vi "Configure Offset and Limits (Reflection Measurement).vi"(0 "VISA resource name":refnum<visa-resource-name>, 1 "Limit Line Value (0 dBm)":dbl, 5 "Line Number (1: Line 1)":i32(ring)=1 items=["Line 1"=1, "Line 2"=2], 9 "Limit Type (0: Upper Line)":i32(ring) items=["Upper Line", "Lower Line"], 11 "error in (no error)":errorcluster) -> (4 "VISA resource name out":refnum<visa-resource-name>, 15 "error out":errorcluster)   [LabVIEW 2022 SP3, in "Agilent N934X Series.lvlib"]
doc: "Configures the general setting for offset and limits of reflection Measurement Option.\n\nNote:\nThis VI is only applicable for N9321C, N9322C, N9323C, N9324C models."
uses:
  <instrlib>/Agilent N934X Series/Agilent N934X Series.lvlib
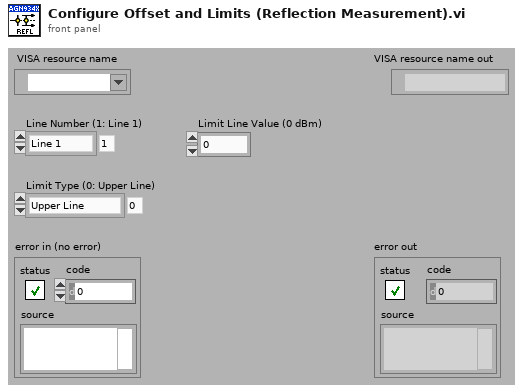
[diagram p1: front panel]
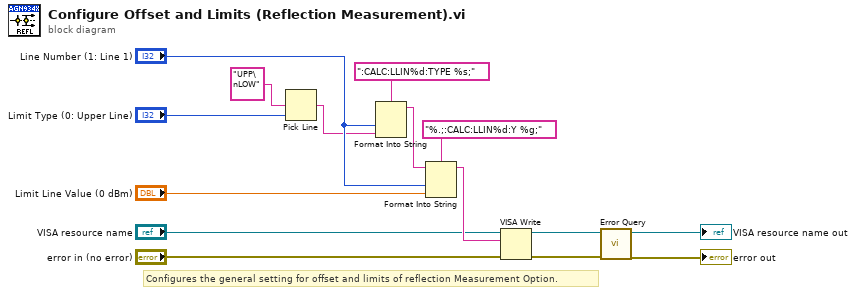
[diagram p0: block diagram]
diagram:
  # "Configures the general setting for offset and limits of reflection Measurement Option."
  n1 = Pick Line(multi-line string="UPP\nLOW", line index="Limit Type (0: Upper Line)") -> (output string=w11:string)  [unwired: 1 in]
  n2 = Format Into String(format string=":CALC:LLIN%d:TYPE %s;", "Line Number (1: Line 1)", w11) -> (resulting string=w10:string)  [unwired: 2 in, 1 out]
  n3 = Format Into String(format string="%.;:CALC:LLIN%d:Y %g;", initial string=w10, "Line Number (1: Line 1)", "Limit Line Value (0 dBm)") -> (resulting string=w7:string)  [unwired: 1 in, 1 out]
  n4 = VISA Write(VISA resource name="VISA resource name", write buffer=w7, error in (no error)="error in (no error)") -> (VISA resource name out=w4:refnum<visa-resource-name>, error out=w3:errorcluster)  [unwired: 1 out]
  n5 = call <instrlib>:"Error Query.vi"("error in (no error)"=w3, "VISA resource name"=w4) -> ("error out"=→"error out":errorcluster, "VISA resource name out"=→"VISA resource name out":refnum<visa-resource-name>)  [unwired: 6 in, 2 out]
